vi "Calibrate Calculate Current Slope and Offset.vi"(0 "VISA resource name":refnum<visa-resource-name>, 1 "Current Measured Low (0)":dbl, 5 "Current Setpoint Low (0)":dbl, 7 "Current Setpoint High (0)":dbl, 9 "Current Measured High (0)":dbl, 11 "error in (no error)":errorcluster) -> (4 "VISA resource name out":refnum<visa-resource-name>, 15 "error out":errorcluster)   [LabVIEW 2018, in "XP Power PLS600.lvlib"]
doc: "Triggers calculation of the specified Current slope and intercept values for the specified conversion. Execution of this command assumes measurements were taken at two distinct points. XP Power suggests 5% and 100% setpoints. \n<b>NOTE</b>: Refer to the power supply user manual's Calibration section for information on the proper sequence of calls. I"
uses:
  XP Power PLS600.lvlib
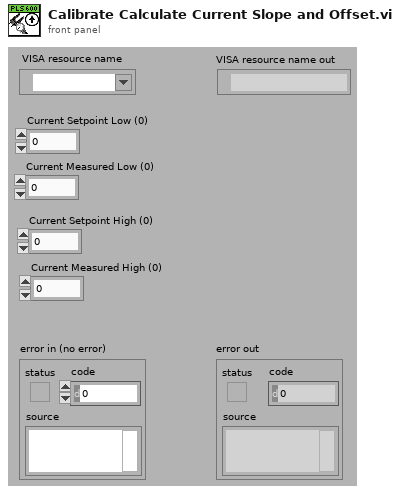
[diagram p1: front panel]
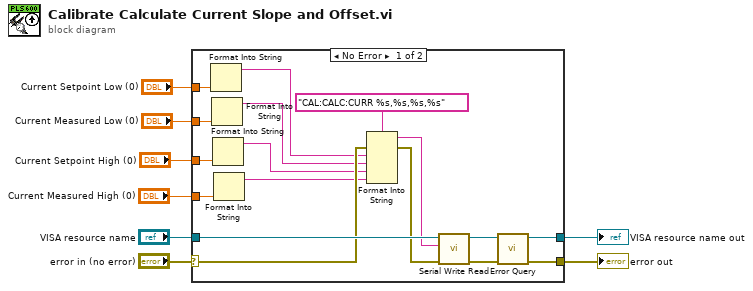
[diagram p0: block diagram]
diagram:
  n1 = case shown="No Error" "error in (no error)" {
    selector: "error in (no error)" -> [w19 w26]
    tunnel: [w25 w27] -> w8
    tunnel: [w24 w26] -> w7
    tunnel: "VISA resource name" -> [w23 w27]
    tunnel: "Current Setpoint Low (0)" -> [w16 _]
    tunnel: "Current Measured Low (0)" -> [w15 _]
    tunnel: "Current Setpoint High (0)" -> [w14 _]
    tunnel: "Current Measured High (0)" -> [w13 _]
    frame No Error {
      n2 = Format Into String(w16) -> (resulting string=w12:string)  [unwired: 3 in, 1 out]
      n3 = Format Into String(w15) -> (resulting string=w11:string)  [unwired: 3 in, 1 out]
      n4 = Format Into String(w14) -> (resulting string=w10:string)  [unwired: 3 in, 1 out]
      n5 = Format Into String(w13) -> (resulting string=w9:string)  [unwired: 3 in, 1 out]
      n6 = Format Into String(format string="CAL:CALC:CURR %s,%s,%s,%s" ("Command to Send"), error in=w19, w12, w11, w10, w9) -> (resulting string=w17:string, error out=w18:errorcluster)  [unwired: 1 in]
      n7 = call "Serial Write Read.vi"("error in (no error)"=w18, "Write Buffer"=w17, "VISA resource name"=w23) -> ("error out"=w21:errorcluster, "VISA resource name out"=w22:refnum<visa-resource-name>)  [unwired: 6 in, 1 out]
      n8 = call "Error Query.vi"("error in (no error)"=w21, "VISA resource name"=w22) -> ("error out"=w24:errorcluster, "VISA resource name out"=w25:refnum<visa-resource-name>)  [unwired: 6 in, 2 out]
    }
    frame Error {
    }
  }
  "VISA resource name out" <- w8
  "error out" <- w7
